vi "Copy Wheel.vi"(8 "error in (no error)":errorcluster, 9 "active wheel indexes in":i32[](array[numeric]), 11 "steering frame ref in":refnum<data-value>) -> (0 "error out":errorcluster, 1 "active wheel indexes out":i32[](array[numeric]), 3 "steering frame ref out":refnum<data-value>, 4 "copied?":bool)   [LabVIEW 2017, in "NI_Robotics_Configure Steering Frame.lvlib"]
uses:
  <vilib>/robotics/Dialog/Configure Steering Frame/NI_Robotics_Configure Steering Frame.lvlib
  <vilib>/robotics/Steering/Steering Frame/NI_Robotics_Steering Frame.lvclass
  <vilib>/robotics/Steering/Steering Frame/NI_Robotics_Steering Frame.lvclass/NI_Robotics_Steering Frame.ctl
  <vilib>/robotics/Steering/Steering Frame/Get Single Wheel in Steering Frame.vi
  <vilib>/robotics/Steering/Steering Frame/Get Multiple Wheels in Steering Frame.vi
  <vilib>/robotics/Steering/Steering Frame/Add Single Wheel to Steering Frame.vi
  <vilib>/robotics/Steering/Wheel/NI_Robotics_Wheel.lvclass
  <vilib>/robotics/Utilities/NI_Robotics Utilities.lvlib
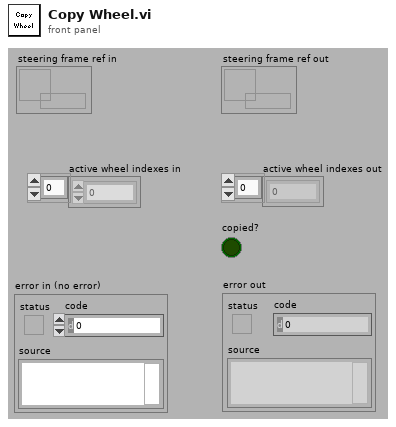
[diagram p1: front panel]
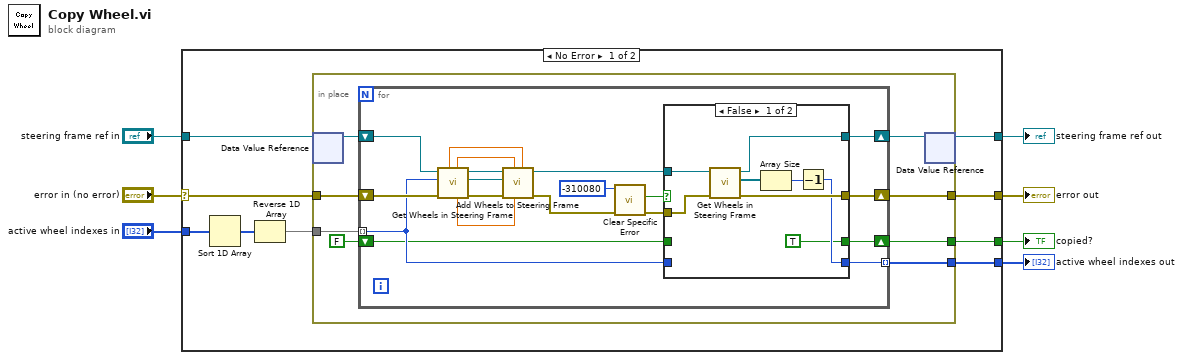
[diagram p0: block diagram]
diagram:
  n1 = case shown="No Error" "error in (no error)" {
    selector: "error in (no error)" -> [w16 w58]
    tunnel: [w15 w58] -> w6
    tunnel: "steering frame ref in" -> [w14 w57]
    tunnel: "active wheel indexes in" -> [w9 w56]
    tunnel: [w13 w57] -> w3
    tunnel: [w12 w56] -> w2
    tunnel: [w11 _] -> w1
    frame No Error {
      n2 = Sort 1D Array(array=w9) -> (sorted array=w10:i32[])
      n3 = Reverse 1D Array(array=w10) -> (reversed array=w8:i32[])
      n4 = in-place {
        in-place-border: w16 -> [w24]
        in-place-border: [w21] -> w15
        in-place-border: w8 -> [w20]
        in-place-border: [w18] -> w12
        in-place-border: [w19] -> w11
        n5 = in-place-dvr #1(w14) -> (w23:refnum<class "NI_Robotics_Steering Frame.lvclass">)  [unwired: 1 out]
        n6 = for {
          tunnel: w20 -> [w28] mode=indexing
          shift-right: [w35] -> w22
          shift-left: w23 -> [w42]
          shift-right: [w34] -> w21
          shift-left: w24 -> [w43]
          tunnel: [w26] -> w18 mode=indexing
          shift-right: [w27] -> w19
          shift-left: FALSE -> [w25]
          n7 = call-poly <vilib>:"Get Wheels in Steering Frame.vi"("error in (no error)"=w43, "wheel index"=w28, "steering frame in"=w42) -> ("error out"=w33:errorcluster, "wheel"=w41:refnum<class "NI_Robotics_Wheel.lvclass">, "steering frame out"=w40:refnum<class "NI_Robotics_Steering Frame.lvclass">, "frame angle (rad)"=w37:dbl, "y position"=w39:dbl, "x position"=w38:dbl)  [unwired: 2 in, 1 out]
          n8 = call-poly <vilib>:"Add Wheels to Steering Frame.vi"("x position"=w38, "frame angle (rad)"=w37, "y position"=w39, "error in (no error)"=w33, "wheel"=w41, "steering frame in"=w40) -> ("error out"=w31:errorcluster, "steering frame out"=w36:refnum<class "NI_Robotics_Steering Frame.lvclass">)  [unwired: 4 in]
          n9 = call <vilib>:"Clear Specific Error.vi"("error in (no error)"=w31, "code"=-310080) -> ("error out"=w29:errorcluster, "cleared?"=w30:bool)  [unwired: 7 in, 1 out]
          n10 = case shown="False" w30 {
            tunnel: w36 -> [w51 w55]
            tunnel: [w50 w55] -> w35
            tunnel: [w49 w54] -> w34
            tunnel: [w46 w53] -> w26
            tunnel: w29 -> [w45 w54]
            tunnel: w28 -> [_ w53]
            tunnel: [TRUE w52] -> w27
            tunnel: w25 -> [_ w52]
            frame False {
              n11 = call-poly <vilib>:"Get Wheels in Steering Frame.vi"("error in (no error)"=w45, "steering frame in"=w51) -> ("error out"=w49:errorcluster, "wheels"=w48:refnum<class "NI_Robotics_Wheel.lvclass">[], "steering frame out"=w50:refnum<class "NI_Robotics_Steering Frame.lvclass">)  [unwired: 3 in, 4 out]
              n12 = Array Size(array=w48) -> (size(s)=w47:i32)
              n13 = Decrement(x=w47) -> (x-1=w46:i32)
            }
            frame True {
            }
          }
        }
        n14 = in-place-dvr #1(w22) -> (w13:refnum<data-value>)  [unwired: 1 out]
      }
    }
    frame Error {
    }
  }
  "error out" <- w6
  "active wheel indexes out" <- w2
  "steering frame ref out" <- w3
  "copied?" <- w1
